vi "atMonochromator_logEvent_SelectedGrating.vi"(8 "error in (no error)":errorcluster, 11 "logevent_SelectedGrating_Ctl":T1) -> (0 "error out":errorcluster, 2 "function return":i32, 3 "logevent_SelectedGrating_Ctl out":T1)   [LabVIEW 2016, in "SALLV_atMonochromator.lvlib"]
doc: "int atMonochromator_shm_logEvent_SelectedGratingLV(atMonochromator_logevent_SelectedGratingLV *logevent_SelectedGrating_Ctl );"
uses:
  SALLV_atMonochromator.lvlib
  DataTypes/logevent_SelectedGrating.ctl
  SALLV_atMonochromator.so
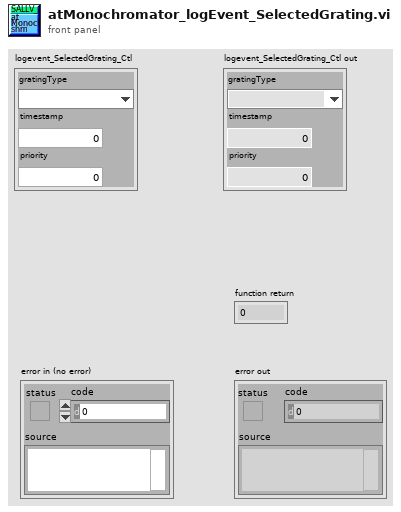
[diagram p1: front panel]
types:
  T1 = typedef "SALLV_atMonochromator.lvlib/logevent_SelectedGrating.ctl" = cluster{"gratingType":enum16{"", "Blue", "Red", "Mirror"}, "timestamp":dbl, "priority":i32}
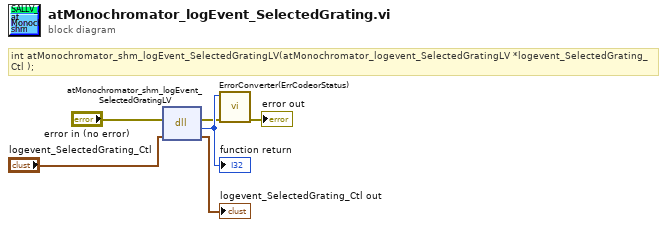
[diagram p0: block diagram]
diagram:
  # "int atMonochromator_shm_logEvent_SelectedGratingLV(atMonochromator_logevent_SelectedGratingLV *logevent_SelectedGrating_Ctl );"
  n1 = dll-call lib="home/andres/Desktop/SAL_atMonochromator/SALLV_atMonochromator.*" fn="atMonochromator_shm_logEvent_SelectedGratingLV"(error in="error in (no error)", "logevent_SelectedGrating_Ctl"="logevent_SelectedGrating_Ctl") -> (error out=w2:errorcluster, w6:i32, "logevent_SelectedGrating_Ctl"=→"logevent_SelectedGrating_Ctl out":T1)  [unwired: 2 in, 1 out]
  "function return" <- w6
  n2 = call "ErrorConverter(ErrCodeorStatus).vi"("error in (no error)"=w2, "error code"=w6) -> ("error out"=→"error out":errorcluster)  [unwired: 9 in]
